vi "Plot.vi"(9 "Position_Goal_Deg":dbl, 10 "Velocity_RadPerSec":dbl, 11 "Position_Deg":dbl) -> (2 "XY Graph":cluster{"Y":dbl[], "Y":dbl[]}[](graph))   [LabVIEW 2023]
uses:
  <vilib>/Rock Robotics/WPI/ThirdParty/JAS_Junk/TrajLib/VI/Util_GetTime_U32.vi
  <vilib>/Rock Robotics/WPI/ThirdParty/JAS_Junk/TrajLib/VI/Util_GetTime_U64.vi
  <vilib>/Rock Robotics/WPI/ThirdParty/JAS_Junk/TrajLib/Trajectory_Library.lvlib
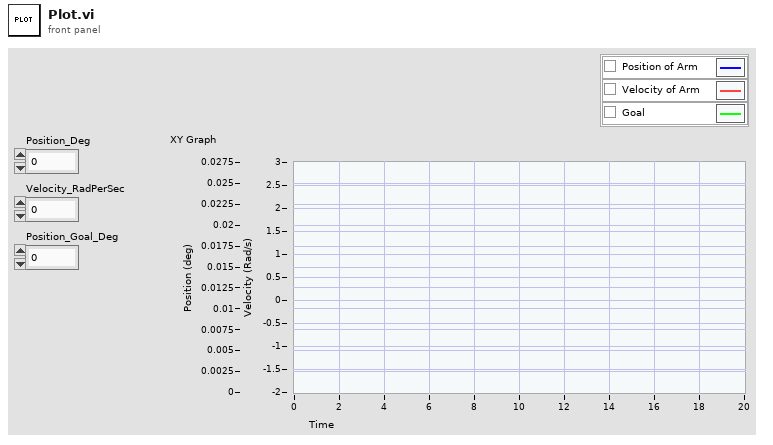
[diagram p1: front panel]
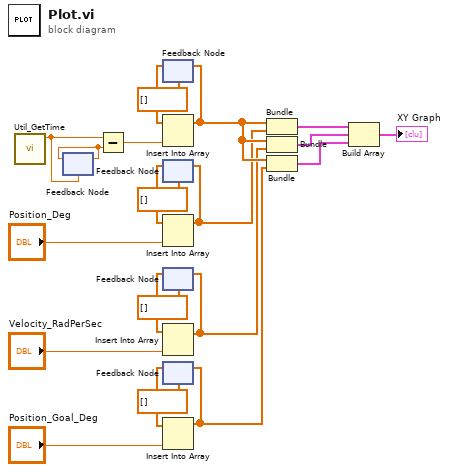
[diagram p0: block diagram]
diagram:
  n1 = call <vilib>:"Util_GetTime.vi"() -> ("FPGA_Time_Seconds"=w1:dbl)  [unwired: 9 in, 2 out]
  n2 = feedback #1(w1) -> (w2:dbl)
  n3 = feedback-in #1(w2) -> ()
  n4 = Subtract(x=w1, y=w2) -> (x-y=w3:dbl)
  n5 = feedback #2(dbl[] []) -> (w4:dbl[])
  n6 = Insert Into Array(array=w4, new element=w3) -> (w18:dbl[])  [unwired: 1 in]
  n7 = feedback-in #2(w18) -> ()
  n8 = feedback #3(dbl[] []) -> (w7:dbl[])
  n9 = Insert Into Array(array=w7, new element="Position_Deg") -> (w10:dbl[])  [unwired: 1 in]
  n10 = feedback-in #3(w10) -> ()
  n11 = feedback #4(dbl[] []) -> (w9:dbl[])
  n12 = Insert Into Array(array=w9, new element="Velocity_RadPerSec") -> (w11:dbl[])  [unwired: 1 in]
  n13 = feedback-in #4(w11) -> ()
  n14 = feedback #5(dbl[] []) -> (w14:dbl[])
  n15 = Insert Into Array(array=w14, new element="Position_Goal_Deg") -> (w16:dbl[])  [unwired: 1 in]
  n16 = feedback-in #5(w16) -> ()
  n17 = Bundle(w18, w10) -> (w12:cluster{dbl[], dbl[]})  [unwired: 1 in]
  n18 = Bundle(w18, w11) -> (w13:cluster{dbl[], dbl[]})  [unwired: 1 in]
  n19 = Bundle(w18, w16) -> (w17:cluster{dbl[], dbl[]})  [unwired: 1 in]
  n20 = Build Array(w12, w13, w17) -> (→"XY Graph":cluster{dbl[], dbl[]}[])
